vi "Server.vi"() -> ()   [LabVIEW 2021, in "Server_Stream.lvlib"]
uses:
  Server_Stream.lvlib
  Demo_server/RPC Service/Communicate/Communicate.lvclass
  <vilib>/gRPC/LabVIEW gRPC Library/Shared/grpcId.ctl
  <vilib>/gRPC/LabVIEW gRPC Servicer/Servicer/Servicer.lvclass/Servicer.ctl
  Demo_server/RPC Service/Communicate/Communicate.lvclass/Communicate.ctl
  Demo_server/RPC Messages/Communication_StreamData.ctl
  <vilib>/numeric/Random Number (Range) U64.vi
  <vilib>/numeric/sub_Random U32.vi
  <vilib>/gRPC/LabVIEW gRPC Servicer/Servicer/Servicer.lvclass
  Demo_server/Demo_server.lvlib
  <vilib>/gRPC/LabVIEW gRPC Library/grpc-lvsupport-release.lvlib
panel:
  in  "Server Address":string="localhost:50051"
  out "Waveform Chart":u64(graph)
  out "Running?":bool
  out "Listening Port":i32
  # "Server Stream Server"
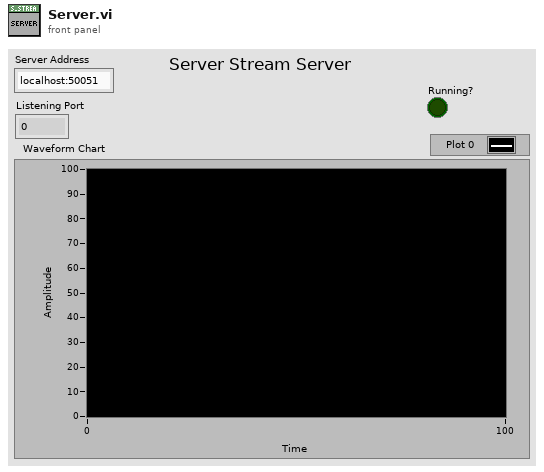
[diagram p1: front panel]
types:
  T1 = typedef "grpc-lvsupport-release.lvlib/grpcId.ctl" = u64
  T2 = cluster{"Running?":bool, "gRPCid out":T1, "Index":i32}
  T3 = typedef "Demo_server.lvlib/Communicate.lvclass/Server gRPC UEs.ctl" = cluster{"Communicate Stream gRPC UE":refnum<user-event>}
  T4 = typedef "Demo_server.lvlib/Communication_StreamData.ctl" = cluster{"data":i32, "Status":bool}
  T5 = typedef "Demo_server.lvlib/Communication_ControlStream.ctl" = cluster{"Start":bool}
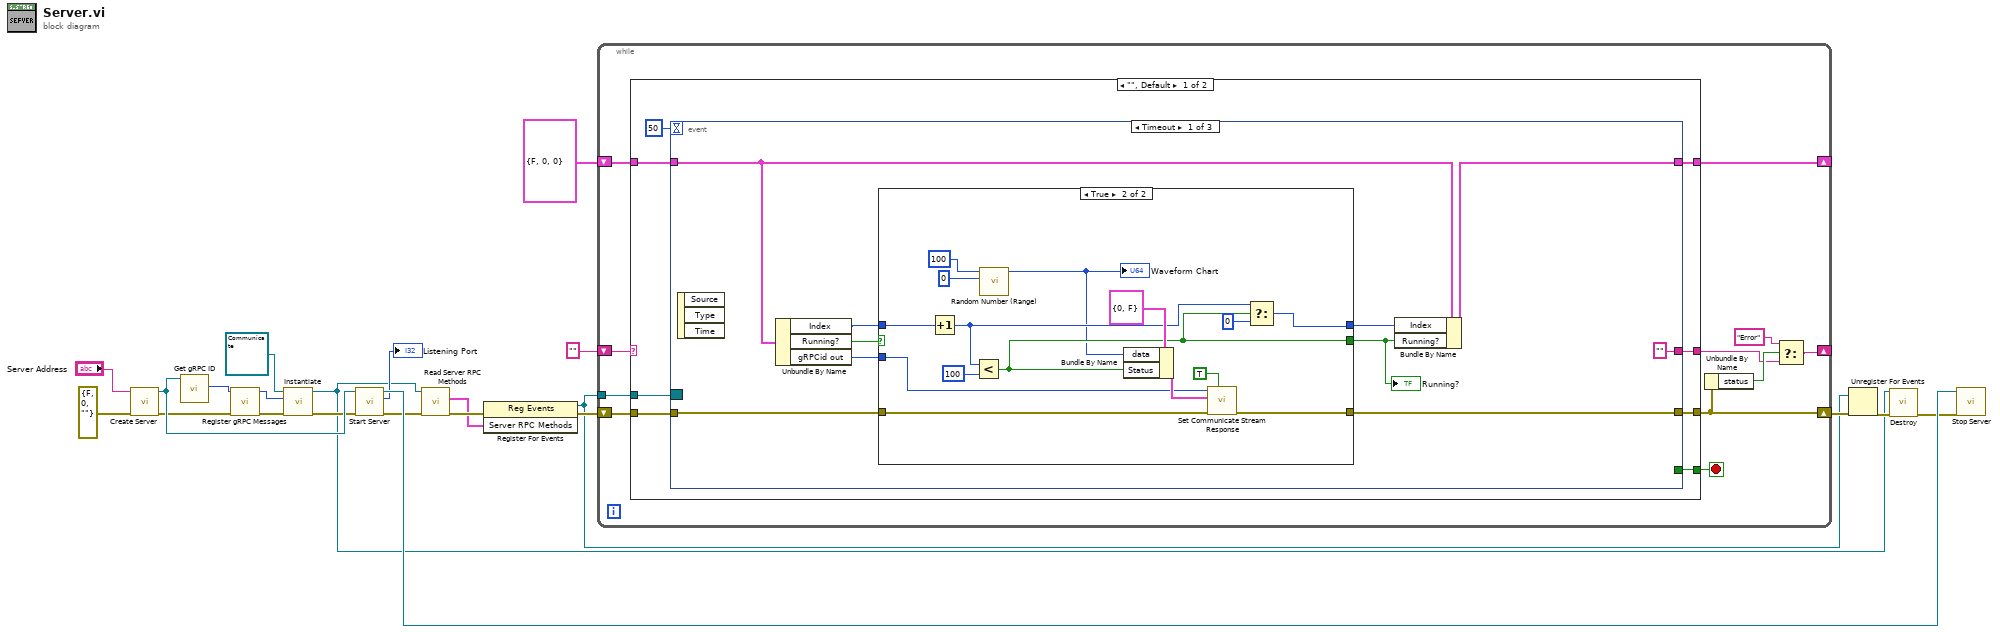
[diagram p0: block diagram]
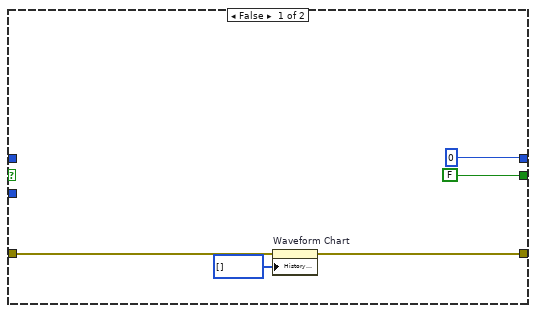
[diagram p2: hidden frame]
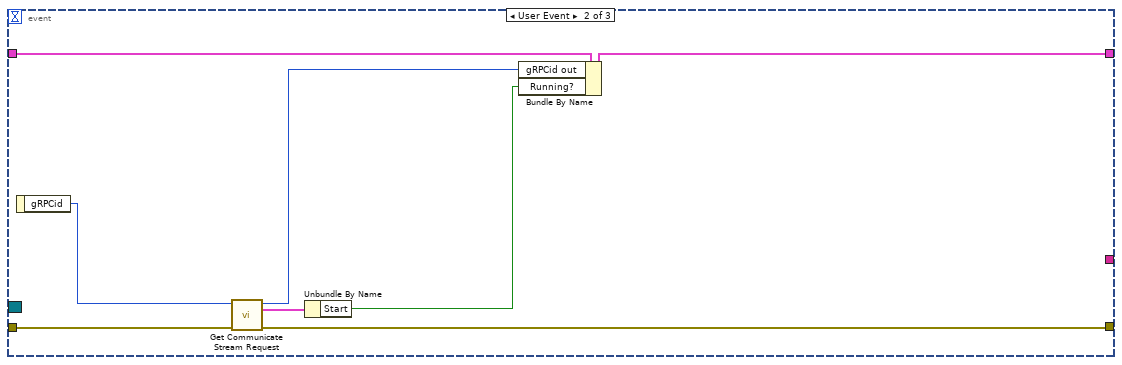
[diagram p3: hidden frame]
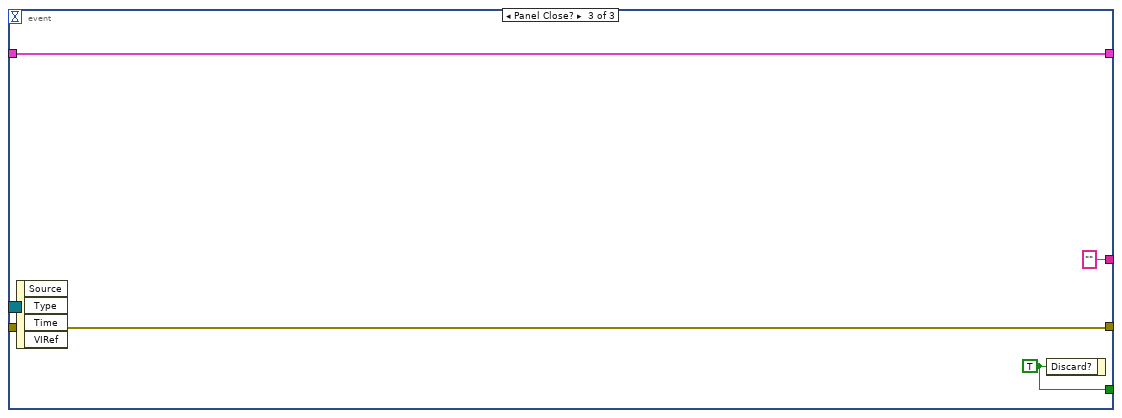
[diagram p4: hidden frame]
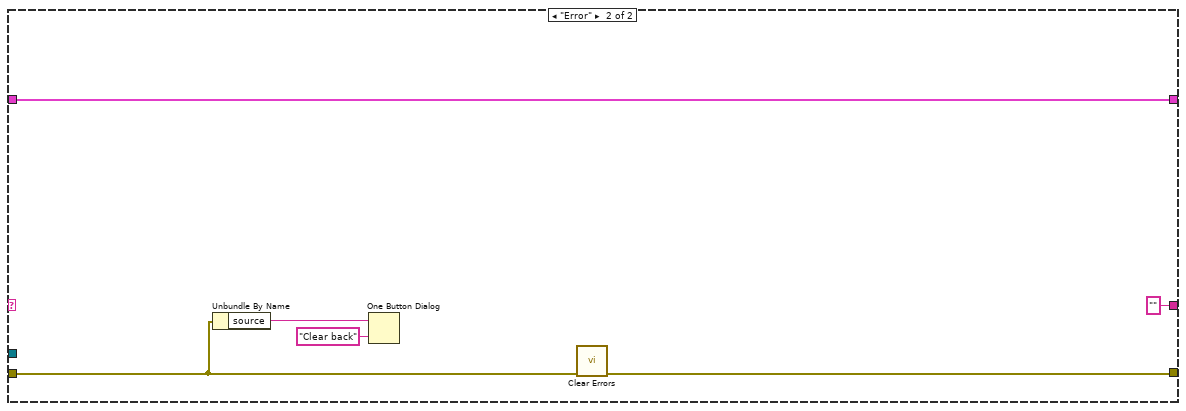
[diagram p5: hidden frame]
diagram:
  n1 = call <vilib>:"Create Server.vi"("error in"=errorcluster {"status"=FALSE, "code"=0, "source"=""} ("error in (no error)"), "Server Address"="Server Address") -> ("error out"=w3:errorcluster, "gRPC Server out"=w14:refnum<class "Servicer.lvclass">)  [unwired: 8 in]
  n2 = call <vilib>:"Get gRPC ID.vi"("OOP Server in"=w14) -> ("gRPC ID"=w4:T1)  [unwired: 9 in, 1 out]
  n3 = call "Register gRPC Messages.vi"("error in (no error)"=w3, "gRPC ID"=w4) -> ("error out"=w2:errorcluster, "gRPC ID Out"=w5:T1)  [unwired: 8 in]
  n4 = call-dynamic "Instantiate.vi"("error in"=w2, "gRPCid"=w5, "iService"=refnum<class "Communicate.lvclass"> refnum ("gRPC Server in")) -> ("error out"=w13:errorcluster, "iService"=w7:refnum<class "Communicate.lvclass">)  [unwired: 7 in]
  n5 = call <vilib>:"Start Server.vi"("error in"=w13, "gRPC Server in"=w14) -> ("error out"=w6:errorcluster, "Listening Port"=→"Listening Port":i32, "gRPC Server out"=w16:refnum<class "Servicer.lvclass">)  [unwired: 7 in]
  n6 = call "Read Server RPC Methods.vi"("error in (no error)"=w6, "SignalGeneratorService in"=w7) -> ("error out"=w9:errorcluster, "Server RPC Methods"=w8:T3)  [unwired: 7 in, 1 out]
  n7 = register-events(error in=w9, w8) -> (reference out=w19:refnum<event-registration>, error out=w21:errorcluster)  [unwired: 1 in]
  n8 = while {
    shift-right: [w30] -> w20
    shift-left: w21 -> [w32]
    shift-right: [w28] -> _
    shift-left: "" -> [w33]
    tunnel: w19 -> [w25]
    shift-right: [w23] -> _
    shift-left: T2 {"Running?"=FALSE, "gRPCid out"=0, "Index"=0} -> [w24]
    stop <- w31 stop-if-true
    n9 = case shown="\"\", Default" w33 {
      tunnel: w32 -> [w41 w88]
      tunnel: [w40 w89] -> w30
      tunnel: [w39 ""] -> w27
      tunnel: [w38 _] -> w31
      tunnel: w25 -> [w36 _]
      tunnel: w24 -> [w35 w84]
      tunnel: [w34 w84] -> w23
      frame "", Default {
        n10 = event shown="[0] Timeout" {
          selector: w36 -> [_ _ _]
          dyn-events: _ -> [_ _ _]
          timeout: 50 -> [_ _ _]
          tunnel: w41 -> [w49 w77 w83]
          tunnel: [w50 w76 w83] -> w40
          tunnel: ["" _ ""] -> w39
          tunnel: [_ _ w81] -> w38
          tunnel: w35 -> [w48 w79 w80]
          tunnel: [w45 w75 w80] -> w34
          event Timeout {
            n11 = event-data() -> ()  [unwired: 1 in, 3 out]
            n12 = Unbundle By Name(w48) -> ("Index"=w46:i32, "Running?"=w42:bool, "gRPCid out"=w47:T1)
            n13 = case shown="True" w42 {
              tunnel: [w54 w71] -> w50
              tunnel: w49 -> [w53 w70]
              tunnel: w47 -> [_ w66]
              tunnel: w46 -> [_ w65]
              tunnel: [0 w61] -> w44
              tunnel: [FALSE w63] -> w43
              frame False {
                n14 = property on="Waveform Chart" class="WFChart (strict)"(error in=w53, "History Data"=u64[] []) -> (error out=w54:errorcluster)  [unwired: 1 in, 1 out]
              }
              frame True {
                n15 = Increment(x=w65) -> (x+1=w62:i32)
                n16 = Less?(x=w62, y=100) -> (x < y?=w63:bool)
                n17 = call-poly <vilib>:"Random Number (Range).vi"("lower bound (0)"=u64 0, "upper bound (100)"=u64 100) -> ("number"=w57:u64)  [unwired: 9 in]
                "Waveform Chart" <- w57
                n18 = Bundle By Name(cluster=T4 {"data"=0, "Status"=FALSE} ("Message Data"), "data"=w57, "Status"=w63) -> (w68:T4)
                n19 = call "Set Communicate Stream Response.vi"("Streaming? (F)"=TRUE, "error in (no error)"=w70, "Message Data"=w68, "gRPCid in"=w66) -> ("error out"=w71:errorcluster)  [unwired: 7 in]
                n20 = Select(t=w62, s=w63, f=0) -> (s? t:f=w61:i32)
              }
            }
            "Running?" <- w43
            n21 = Bundle By Name(cluster=w48, "Index"=w44, "Running?"=w43) -> (w45:T2)
          }
          event User Event {
            n22 = event-data() -> ("gRPCid"=w78:T1)  [unwired: 1 in]
            n23 = call "Get Communicate Stream Request.vi"("error in (no error)"=w77, "gRPCid in"=w78) -> ("error out"=w76:errorcluster, "Message Data"=w73:T5, "gRPCid out"=w74:T1)  [unwired: 7 in]
            n24 = Unbundle By Name(w73) -> ("Start"=w72:bool)
            n25 = Bundle By Name(cluster=w79, "gRPCid out"=w74, "Running?"=w72) -> (w75:T2)
          }
          event Panel Close? {
            w81 = TRUE ("Discard?")
            n26 = event-data() -> ()  [unwired: 1 in, 4 out]
            n27 = event-data("Discard?"=w81) -> ()  [unwired: 1 in, 1 out]
          }
        }
      }
      frame "Error" {
        n28 = Unbundle By Name(w88) -> ("source"=w86:string)
        n29 = One Button Dialog(message=w86, button name ("OK")="Clear back") -> ()  [unwired: 1 out]
        n30 = call <vilib>:"Clear Errors.vi"("error in (no error)"=w88) -> ("error out"=w89:errorcluster)  [unwired: 5 in, 1 out]
      }
    }
    n31 = Unbundle By Name(w30) -> ("status"=w29:bool)
    n32 = Select(t="Error", s=w29, f=w27) -> (s? t:f=w28:string)
  }
  n33 = Unregister For Events(event registration refnum=w19, error in=w20) -> (error out=w11:errorcluster)
  n34 = call-dynamic "Destroy.vi"("error in (no error)"=w11, "SignalGeneratorService in"=w7) -> ("error out"=w12:errorcluster)  [unwired: 8 in, 1 out]
  n35 = call <vilib>:"Stop Server.vi"("error in"=w12, "gRPC Server in"=w16) -> ()  [unwired: 9 in, 1 out]
